vi "LM Three Asymmetric Gaussians and gradient.vi"(3 "output control":T1, 4 "data":variant, 5 "X":dbl[](array[numeric]), 6 "a":dbl[](array[numeric])) -> (0 "error out":errorcluster, 1 "f'(X,a)":dbl[][](array[numeric]), 2 "f(X,a)":dbl[](array[numeric]))   [LabVIEW 2021, in "Fits.lvlib"]
doc: "This template is the starting point for creating a model function to be passed to the Nonlinear Curve Fit.vi."
uses:
  Fits.lvlib
  <vilib>/gmath/NumericalOptimization/LM_output select.ctl
  D-Only Fixed Parameters.ctl
  <vilib>/gmath/NI_Gmath.lvlib
panel:
  # "Parameters:\n\namplitude 1: A1\ncenter 1: t1\nSDV 1-: s1-\nSDV 1+: s1+\nAmplitude 2: A2\ncenter 2: t2\nSDV 2-: s2-\nSDV 2+: s2+\nAmplitude 3: A3\ncenter 3: t3\nSDV 3-: s3-\nSDV 3+: s3+"
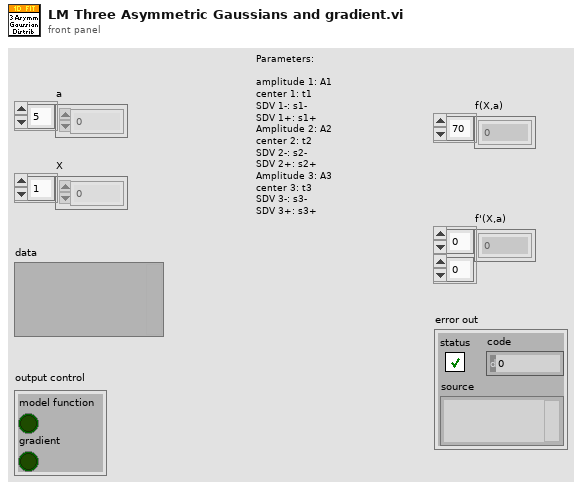
[diagram p1: front panel]
types:
  T1 = typedef "NI_Gmath.lvlib/LM_output select.ctl" = cluster{"model function":bool, "gradient":bool}
  T2 = typedef "Fits.lvlib/D-Only Fixed Parameters.ctl" = cluster{"Fix D-only Peak Location":bool, "Peak Location":dbl, "Fix D-only Peak FWHM":bool, "Peak FWHM":dbl}
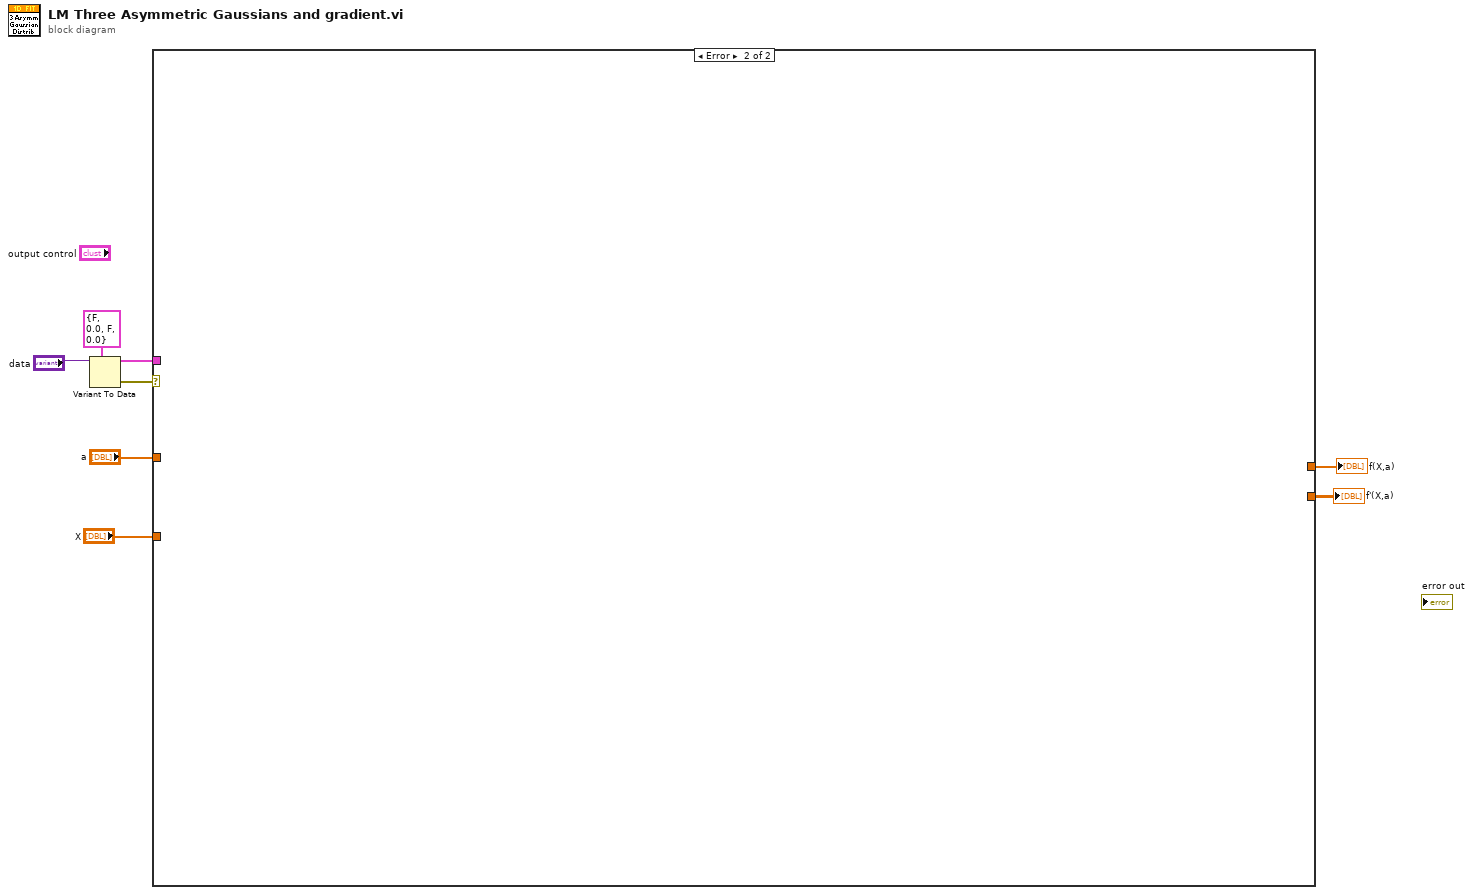
[diagram p0: block diagram]
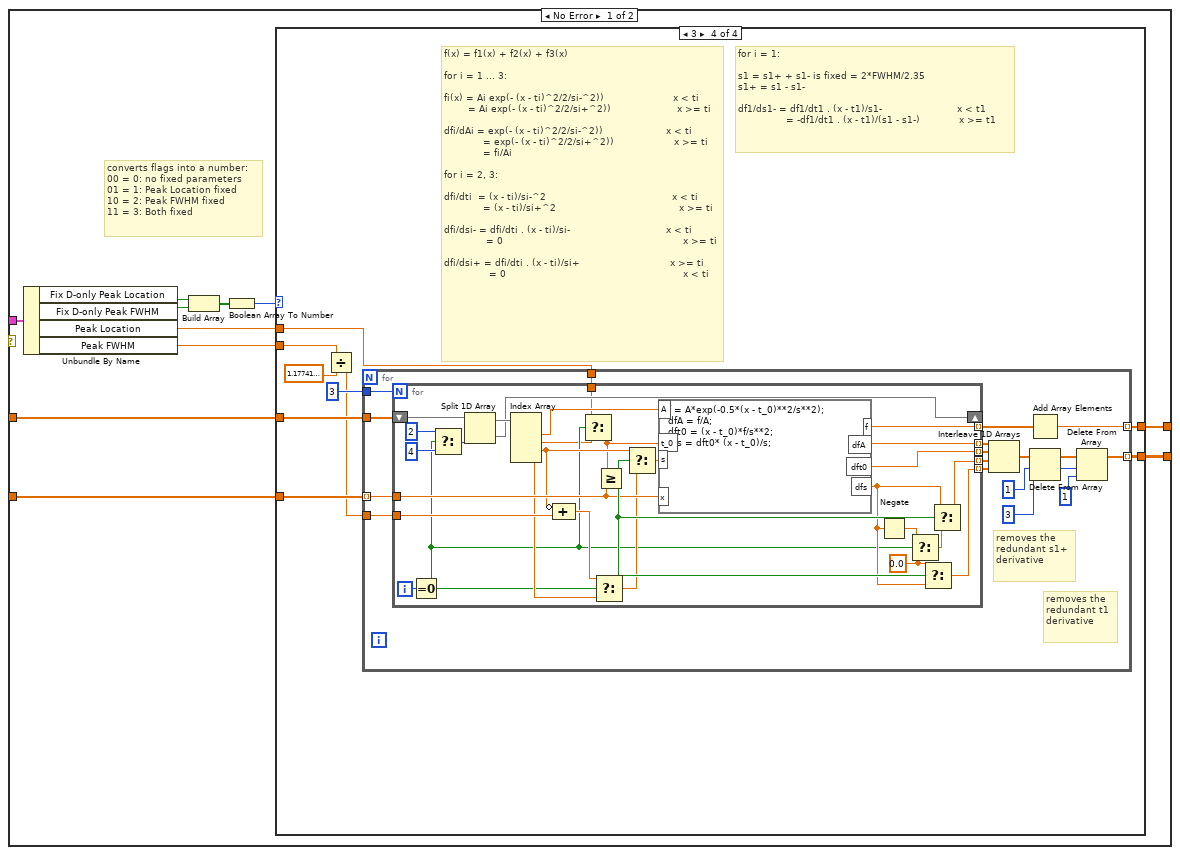
[diagram p2: hidden frame]
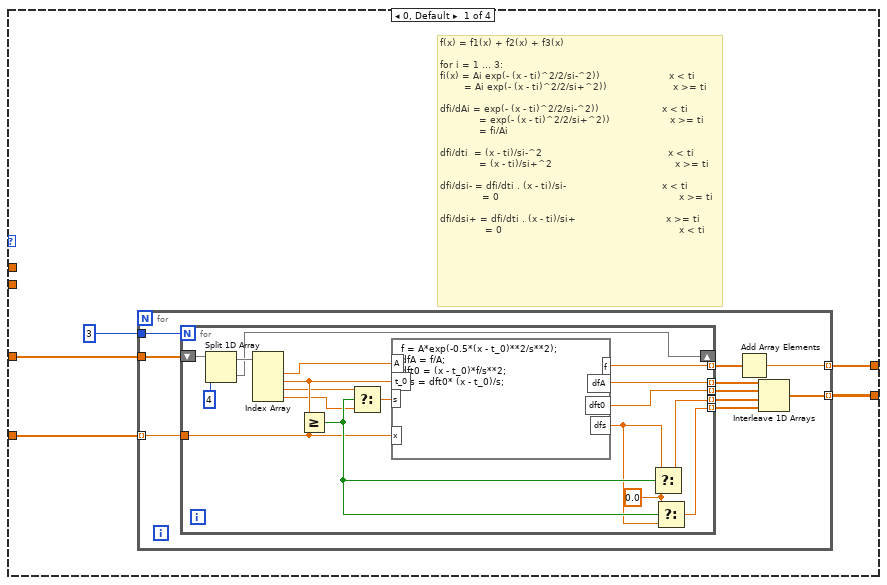
[diagram p3: hidden frame]
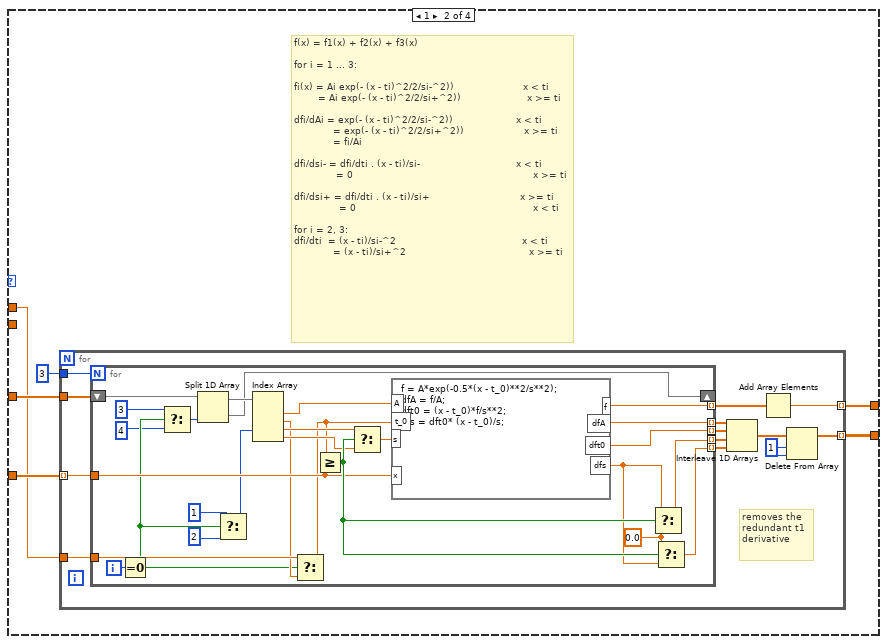
[diagram p4: hidden frame]
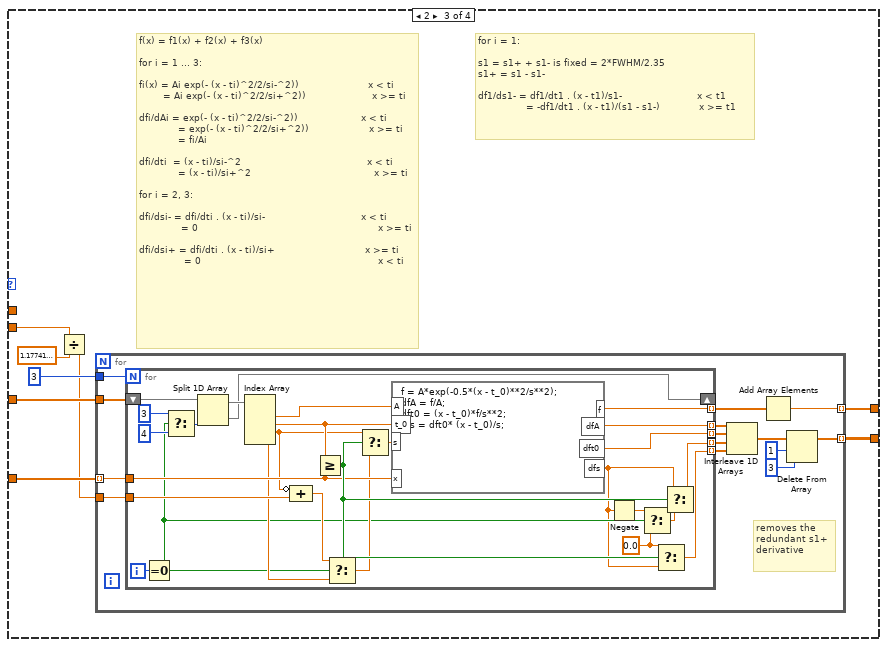
[diagram p5: hidden frame]
diagram:
  n1 = Variant To Data(type=T2 {"Fix D-only Peak Location"=FALSE, "Peak Location"=0.0, "Fix D-only Peak FWHM"=FALSE, "Peak FWHM"=0.0} ("Fixed Parameters"), Variant="data") -> (data=w2:T2, error out=w3:errorcluster)  [unwired: 1 in]
  n2 = case shown="Error" w3 {
    tunnel: "a" -> [w19 _]
    tunnel: "X" -> [w18 _]
    tunnel: [w17 _] -> w1
    tunnel: [w16 _] -> w6
    tunnel: w2 -> [w12 _]
    frame No Error {
      # "converts flags into a number:\n00 = 0: no fixed parameters\n01 = 1: Peak Location fixed\n10 = 2: Peak FWHM fixed\n11 = 3: Both fixed"
      n3 = Unbundle By Name(w12) -> ("Fix D-only Peak Location"=w15:bool, "Fix D-only Peak FWHM"=w14:bool, "Peak Location"=w10:dbl, "Peak FWHM"=w9:dbl)
      n4 = Build Array(w15, w14) -> (w13:bool[])
      n5 = Boolean Array To Number(Boolean array=w13) -> (number=w11:u32)
      n6 = case shown="3" w11 {
        tunnel: w19 -> [w20 w54 w102 w152]
        tunnel: w18 -> [w24 w58 w106 w156]
        tunnel: [w23 w57 w105 w155] -> w17
        tunnel: [w22 w56 w104 w154] -> w16
        tunnel: w10 -> [_ w53 _ w148]
        tunnel: w9 -> [_ _ w100 w150]
        frame 0, Default {
          # "f(x) = f1(x) + f2(x) + f3(x)\n\nfor i = 1 ... 3: \nfi(x) = Ai exp(- (x - ti)^2/2/si-^2))                       x < ti\n        = Ai exp(- (x - ti)^2/2/si+^2))                      x >= ti\n\ndfi/dAi = exp(- (x - ti)^2/2/si-^2))                     x < ti\n             = exp(- (x - ti)^2/2/si+^2))                    x >= ti\n             = fi/Ai\n\ndfi/dti  = (x - ti)/si-^2                                          x < ti\n             = (x - ti)/si+^2                                         x >= ti\n\ndfi/dsi- = dfi/dti . (x - ti)/si-                                x < ti\n              = 0                                                            x >= ti\n\ndfi/dsi+ = dfi/dti . (x - ti)/si+                              x >= ti\n               = 0                                                           x < ti"
          n7 = for {
            tunnel: w24 -> [w34] mode=indexing
            tunnel: [w30] -> w23 mode=indexing
            tunnel: [w25] -> w22 mode=indexing
            tunnel: 3 -> [w32]
            tunnel: w20 -> [w31]
            n8 = for {
              N: w32 -> [_]
              tunnel: [w48] -> w29 mode=indexing
              tunnel: [w47] -> w33 mode=indexing
              tunnel: [w46] -> w28 mode=indexing
              tunnel: [w45] -> w27 mode=indexing
              tunnel: [w44] -> w26 mode=indexing
              tunnel: w34 -> [w43]
              shift-right: [w35] -> _
              shift-left: w31 -> [w42]
              w50 = 0.0 ("f")
              n9 = Split 1D Array(array=w42, index=4) -> (first subarray=w40:dbl[], second subarray=w35:dbl[])
              n10 = Index Array(array=w40) -> (element #1=w39:dbl, element #2=w38:dbl, element #3=w37:dbl, element #4=w36:dbl)  [unwired: 4 in]
              n11 = Greater Or Equal?(x=w38, y=w43) -> (x >= y?=w51:bool)
              n12 = Select(t=w37, s=w51, f=w36) -> (s? t:f=w52:dbl)
              n13 = formula code="f = A*exp(-0.5*(x - t_0)**2/s**2);\ndfA = f/A;\ndft0 = (x - t_0)*f/s**2;\ndfs = dft0* (x - t_0)/s;"("A"=w39, "t_0"=w38, "s"=w52, "x"=w43) -> ("f"=w47:dbl, "dfA"=w48:dbl, "dft0"=w46:dbl, "dfs"=w49:dbl)
              n14 = Select(t=w49, s=w51, f=w50) -> (s? t:f=w45:dbl)
              n15 = Select(t=w50, s=w51, f=w49) -> (s? t:f=w44:dbl)
            }
            n16 = Add Array Elements(numeric array=w33) -> (sum=w30:dbl)
            n17 = Interleave 1D Arrays(w29, w28, w27, w26) -> (w25:dbl[])
          }
        }
        frame 1 {
          # "f(x) = f1(x) + f2(x) + f3(x)\n\nfor i = 1 ... 3: \n\nfi(x) = Ai exp(- (x - ti)^2/2/si-^2))                       x < ti\n        = Ai exp(- (x - ti)^2/2/si+^2))                      x >= ti\n\ndfi/dAi = exp(- (x - ti)^2/2/si-^2))                     x < ti\n             = exp(- (x - ti)^2/2/si+^2))                    x >= ti\n             = fi/Ai\n\ndfi/dsi- = dfi/dti . (x - ti)/si-                                x < ti\n              = 0                                                            x >= ti\n\ndfi/dsi+ = dfi/dti . (x - ti)/si+                              x >= ti\n               = 0                                                           x < ti\n\nfor i = 2, 3:\ndfi/dti  = (x - ti)/si-^2                                          x < ti\n             = (x - ti)/si+^2                                         x >= ti"
          n18 = for {
            tunnel: w58 -> [w71] mode=indexing
            tunnel: [w67] -> w57 mode=indexing
            tunnel: [w60] -> w56 mode=indexing
            tunnel: 3 -> [w69]
            tunnel: w54 -> [w68]
            tunnel: w53 -> [w61]
            w59 = 1 ("length")
            # "removes the redundant t1 derivative"
            n19 = for {
              N: w69 -> [_]
              tunnel: [w94] -> w66 mode=indexing
              tunnel: [w93] -> w70 mode=indexing
              tunnel: [w92] -> w65 mode=indexing
              tunnel: [w91] -> w64 mode=indexing
              tunnel: [w90] -> w63 mode=indexing
              tunnel: w71 -> [w89]
              shift-right: [w83] -> _
              shift-left: w68 -> [w88]
              tunnel: w61 -> [w81]
              i -> [w82]
              w96 = 0.0 ("f")
              n20 = Equal To 0?(x=w82) -> (x = 0?=w75:bool)
              n21 = Select(t=3, s=w75, f=4 ("index")) -> (s? t:f=w72:i32)
              n22 = Split 1D Array(array=w88, index=w72) -> (first subarray=w87:dbl[], second subarray=w83:dbl[])
              n23 = Select(t=1, s=w75, f=2 ("index")) -> (s? t:f=w78:i32)
              n24 = Index Array(array=w87, index #3=w78) -> (element #1=w86:dbl, element #2=w80:dbl, element #3=w85:dbl, element #4=w84:dbl)  [unwired: 3 in]
              n25 = Select(t=w81, s=w75, f=w80) -> (s? t:f=w79:dbl)
              n26 = Greater Or Equal?(x=w79, y=w89) -> (x >= y?=w97:bool)
              n27 = Select(t=w85, s=w97, f=w84) -> (s? t:f=w98:dbl)
              n28 = formula code="f = A*exp(-0.5*(x - t_0)**2/s**2);\ndfA = f/A;\ndft0 = (x - t_0)*f/s**2;\ndfs = dft0* (x - t_0)/s;"("A"=w86, "t_0"=w79, "s"=w98, "x"=w89) -> ("f"=w93:dbl, "dfA"=w94:dbl, "dft0"=w92:dbl, "dfs"=w95:dbl)
              n29 = Select(t=w95, s=w97, f=w96) -> (s? t:f=w91:dbl)
              n30 = Select(t=w96, s=w97, f=w95) -> (s? t:f=w90:dbl)
            }
            n31 = Interleave 1D Arrays(w66, w65, w64, w63) -> (w62:dbl[])
            n32 = Add Array Elements(numeric array=w70) -> (sum=w67:dbl)
            n33 = Delete From Array(array=w62, length=w59, index=w59) -> (array with subset deleted=w60:dbl[])  [unwired: 1 out]
          }
        }
        frame 2 {
          # "for i = 1: \n\ns1 = s1+ + s1- is fixed = 2*FWHM/2.35\ns1+ = s1 - s1-\n\ndf1/ds1- = df1/dt1 . (x - t1)/s1-                         x < t1\n                = -df1/dt1 . (x - t1)/(s1 - s1-)             x >= t1"
          # "f(x) = f1(x) + f2(x) + f3(x)\n\nfor i = 1 ... 3: \n\nfi(x) = Ai exp(- (x - ti)^2/2/si-^2))                       x < ti\n        = Ai exp(- (x - ti)^2/2/si+^2))                      x >= ti\n\ndfi/dAi = exp(- (x - ti)^2/2/si-^2))                     x < ti\n             = exp(- (x - ti)^2/2/si+^2))                    x >= ti\n             = fi/Ai\n\ndfi/dti  = (x - ti)/si-^2                                          x < ti\n             = (x - ti)/si+^2                                         x >= ti\n\nfor i = 2, 3:\n\ndfi/dsi- = dfi/dti . (x - ti)/si-                                x < ti\n              = 0                                                            x >= ti\n\ndfi/dsi+ = dfi/dti . (x - ti)/si+                              x >= ti\n               = 0                                                           x < ti"
          n34 = Divide(x=w100, y=1.1774100225154747) -> (x/y=w99:dbl)
          n35 = for {
            tunnel: w106 -> [w120] mode=indexing
            tunnel: [w116] -> w105 mode=indexing
            tunnel: [w110] -> w104 mode=indexing
            tunnel: 3 -> [w118]
            tunnel: w102 -> [w117]
            tunnel: w99 -> [w107]
            # "removes the redundant s1+ derivative"
            n36 = for {
              N: w118 -> [_]
              tunnel: [w145] -> w115 mode=indexing
              tunnel: [w144] -> w119 mode=indexing
              tunnel: [w143] -> w114 mode=indexing
              tunnel: [w142] -> w113 mode=indexing
              tunnel: [w141] -> w112 mode=indexing
              tunnel: w120 -> [w140]
              shift-right: [w136] -> _
              shift-left: w117 -> [w139]
              tunnel: w107 -> [w132]
              i -> [w135]
              w124 = 0.0 ("f")
              n37 = Equal To 0?(x=w135) -> (x = 0?=w125:bool)
              n38 = Select(t=3, s=w125, f=4 ("index")) -> (s? t:f=w126:i32)
              n39 = Split 1D Array(array=w139, index=w126) -> (first subarray=w138:dbl[], second subarray=w136:dbl[])
              n40 = Index Array(array=w138) -> (element #1=w137:dbl, element #2=w134:dbl, element #3=w133:dbl, element #4=w130:dbl)  [unwired: 4 in]
              n41 = Compound Arithmetic op=ADD(invert w133, w132) -> (w131:dbl)
              n42 = Greater Or Equal?(x=w134, y=w140) -> (x >= y?=w146:bool)
              n43 = Select(t=w131, s=w125, f=w130) -> (s? t:f=w129:dbl)
              n44 = Select(t=w133, s=w146, f=w129) -> (s? t:f=w147:dbl)
              n45 = formula code="f = A*exp(-0.5*(x - t_0)**2/s**2);\ndfA = f/A;\ndft0 = (x - t_0)*f/s**2;\ndfs = dft0* (x - t_0)/s;"("A"=w137, "t_0"=w134, "s"=w147, "x"=w140) -> ("f"=w144:dbl, "dfA"=w145:dbl, "dft0"=w143:dbl, "dfs"=w122:dbl)
              n46 = Negate(x=w122) -> (-x=w121:dbl)
              n47 = Select(t=w121, s=w125, f=w124) -> (s? t:f=w123:dbl)
              n48 = Select(t=w124, s=w146, f=w122) -> (s? t:f=w141:dbl)
              n49 = Select(t=w122, s=w146, f=w123) -> (s? t:f=w142:dbl)
            }
            n50 = Interleave 1D Arrays(w115, w114, w113, w112) -> (w111:dbl[])
            n51 = Add Array Elements(numeric array=w119) -> (sum=w116:dbl)
            n52 = Delete From Array(array=w111, length=1, index=3) -> (array with subset deleted=w110:dbl[])  [unwired: 1 out]
          }
        }
        frame 3 {
          # "for i = 1: \n\ns1 = s1+ + s1- is fixed = 2*FWHM/2.35\ns1+ = s1 - s1-\n\ndf1/ds1- = df1/dt1 . (x - t1)/s1-                         x < t1\n                = -df1/dt1 . (x - t1)/(s1 - s1-)             x >= t1"
          # "f(x) = f1(x) + f2(x) + f3(x)\n\nfor i = 1 ... 3: \n\nfi(x) = Ai exp(- (x - ti)^2/2/si-^2))                       x < ti\n        = Ai exp(- (x - ti)^2/2/si+^2))                      x >= ti\n\ndfi/dAi = exp(- (x - ti)^2/2/si-^2))                     x < ti\n             = exp(- (x - ti)^2/2/si+^2))                    x >= ti\n             = fi/Ai\n\nfor i = 2, 3:\n\ndfi/dti  = (x - ti)/si-^2                                          x < ti\n             = (x - ti)/si+^2                                         x >= ti\n\ndfi/dsi- = dfi/dti . (x - ti)/si-                                x < ti\n              = 0                                                            x >= ti\n\ndfi/dsi+ = dfi/dti . (x - ti)/si+                              x >= ti\n               = 0                                                           x < ti"
          n53 = Divide(x=w150, y=1.1774100225154747) -> (x/y=w149:dbl)
          n54 = for {
            tunnel: w156 -> [w173] mode=indexing
            tunnel: [w169] -> w155 mode=indexing
            tunnel: [w159] -> w154 mode=indexing
            tunnel: 3 -> [w171]
            tunnel: w152 -> [w170]
            tunnel: w149 -> [w161]
            tunnel: w148 -> [w160]
            w158 = 1 ("length")
            # "removes the redundant t1 derivative"
            # "removes the redundant s1+ derivative"
            n55 = for {
              N: w171 -> [_]
              tunnel: [w200] -> w168 mode=indexing
              tunnel: [w199] -> w172 mode=indexing
              tunnel: [w198] -> w167 mode=indexing
              tunnel: [w197] -> w166 mode=indexing
              tunnel: [w196] -> w165 mode=indexing
              tunnel: w173 -> [w195]
              shift-right: [w191] -> _
              shift-left: w170 -> [w194]
              tunnel: w161 -> [w188]
              tunnel: w160 -> [w176]
              i -> [w190]
              w181 = 0.0 ("f")
              n56 = Equal To 0?(x=w190) -> (x = 0?=w177:bool)
              n57 = Select(t=2, s=w177, f=4 ("index")) -> (s? t:f=w182:i32)
              n58 = Split 1D Array(array=w194, index=w182) -> (first subarray=w193:dbl[], second subarray=w191:dbl[])
              n59 = Index Array(array=w193) -> (element #1=w192:dbl, element #2=w174:dbl, element #3=w189:dbl, element #4=w186:dbl)  [unwired: 4 in]
              n60 = Compound Arithmetic op=ADD(invert w189, w188) -> (w187:dbl)
              n61 = Select(t=w176, s=w177, f=w174) -> (s? t:f=w175:dbl)
              n62 = Select(t=w187, s=w177, f=w186) -> (s? t:f=w185:dbl)
              n63 = Greater Or Equal?(x=w175, y=w195) -> (x >= y?=w201:bool)
              n64 = Select(t=w189, s=w201, f=w185) -> (s? t:f=w202:dbl)
              n65 = formula code="f = A*exp(-0.5*(x - t_0)**2/s**2);\ndfA = f/A;\ndft0 = (x - t_0)*f/s**2;\ndfs = dft0* (x - t_0)/s;"("A"=w192, "t_0"=w175, "s"=w202, "x"=w195) -> ("f"=w199:dbl, "dfA"=w200:dbl, "dft0"=w198:dbl, "dfs"=w179:dbl)
              n66 = Negate(x=w179) -> (-x=w178:dbl)
              n67 = Select(t=w178, s=w177, f=w181) -> (s? t:f=w180:dbl)
              n68 = Select(t=w181, s=w201, f=w179) -> (s? t:f=w196:dbl)
              n69 = Select(t=w179, s=w201, f=w180) -> (s? t:f=w197:dbl)
            }
            n70 = Interleave 1D Arrays(w168, w167, w166, w165) -> (w164:dbl[])
            n71 = Add Array Elements(numeric array=w172) -> (sum=w169:dbl)
            n72 = Delete From Array(array=w164, length=w158, index=3) -> (array with subset deleted=w163:dbl[])  [unwired: 1 out]
            n73 = Delete From Array(array=w163, length=w158, index=1) -> (array with subset deleted=w159:dbl[])  [unwired: 1 out]
          }
        }
      }
    }
    frame Error {
    }
  }
  "f(X,a)" <- w1
  "f'(X,a)" <- w6
